vi "sync.wait_on_acknowledgement.vi"(6 "timeout (10s)":dbl=10.0, 8 "error in (no error)":errorcluster, 11 "synchronization in":refnum<class "synchronization.lvclass">) -> (0 "error out":errorcluster, 3 "synchronization out":refnum<class "synchronization.lvclass">)   [LabVIEW 2020, in "synchronization.lvclass"]
uses:
  synchronization.lvclass
  synchronization.lvclass/synchronization.ctl
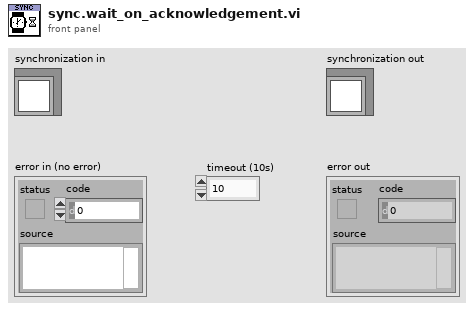
[diagram p1: front panel]
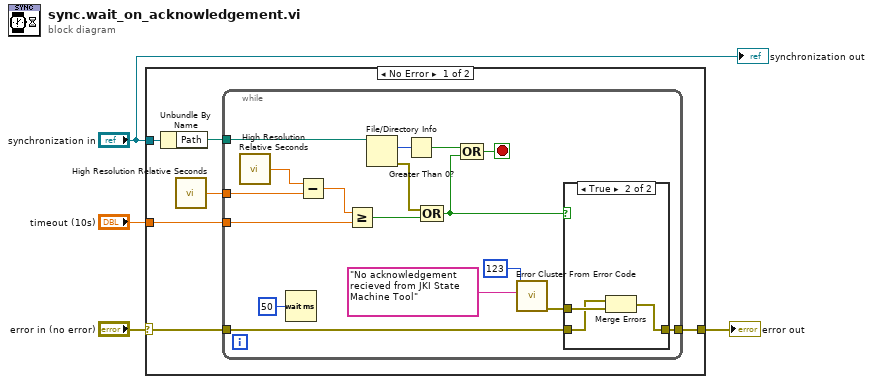
[diagram p0: block diagram]
diagram:
  n1 = case shown="No Error" "error in (no error)" {
    selector: "error in (no error)" -> [w7 w32]
    tunnel: "timeout (10s)" -> [w8 _]
    tunnel: [w6 w32] -> w2
    tunnel: "synchronization in" -> [w5 _]
    frame No Error {
      n2 = Unbundle By Name(w5) -> ("Path"=w10:path)
      n3 = call <vilib>:"High Resolution Relative Seconds.vi"() -> ("relative seconds"=w9:dbl)
      n4 = while {
        tunnel: w10 -> [w26]
        tunnel: w9 -> [w23]
        tunnel: w8 -> [w21]
        tunnel: w7 -> [w13]
        tunnel: [w12] -> w6
        stop <- w15 stop-if-true
        n5 = call <vilib>:"High Resolution Relative Seconds.vi"() -> ("relative seconds"=w24:dbl)
        n6 = Wait (ms)(milliseconds to wait=u32 50) -> ()  [unwired: 1 out]
        n7 = Subtract(x=w24, y=w23) -> (x-y=w22:dbl)
        n8 = Greater Or Equal?(x=w22, y=w21) -> (x >= y?=w17:bool)
        n9 = File/Directory Info(path=w26) -> (size=w25:i64, error out=w20:errorcluster)  [unwired: 1 in, 5 out]
        n10 = Greater Than 0?(x=w25) -> (x > 0?=w16:bool)
        n11 = Compound Arithmetic op=OR(w20, w17) -> (w11:bool)
        n12 = Compound Arithmetic op=OR(w16, w11) -> (w15:bool)
        n13 = call <vilib>:"Error Cluster From Error Code.vi"("error message (\"\")"="No acknowledgement recieved from JKI State Machine Tool" ("error message (\"\")"), "error code (0)"=123) -> ("error out"=w14:errorcluster)  [unwired: 7 in]
        n14 = case shown="True" w11 {
          tunnel: w14 -> [_ w31]
          tunnel: w13 -> [w28 w30]
          tunnel: [w28 w29] -> w12
          frame False {
          }
          frame True {
            n15 = Merge Errors(w30, w31) -> (w29:errorcluster)
          }
        }
      }
    }
    frame Error {
    }
  }
  "error out" <- w2
  "synchronization out" <- "synchronization in"
